vi "Set Convolution Kernel 32f.vi"(8 "Error In":errorcluster, 10 "Kernel In":sgl[][][](array[numeric]), 11 "Convolution Object":T1 {"Convolved Memory Object"."Dimension"."Width" min=1; "Convolved Memory Object"."Dimension"."Height" min=1; "Convolved Memory Object"."Dimension"."Depth" min=1; "Kernel Memory Object"."Dimension"."Width" min=1; "Kernel Memory Object"."Dimension"."Height" min=1; "Kernel Memory Object"."Dimension"."Depth" min=1}) -> (0 "Error Out":errorcluster, 3 "Convolution Object Out":T1 {"Convolved Memory Object"."Dimension"."Width" min=1; "Convolved Memory Object"."Dimension"."Height" min=1; "Convolved Memory Object"."Dimension"."Depth" min=1; "Kernel Memory Object"."Dimension"."Width" min=1; "Kernel Memory Object"."Dimension"."Height" min=1; "Kernel Memory Object"."Dimension"."Depth" min=1})   [LabVIEW 2012, in "OpenCLV x64.lvlib"]
doc: "Creates and copies a convolution kernel from Labview to the device. The convolution kernel should have have {N - 2, N - 2, N - 2} dimensions than the target memory being convolved."
uses:
  OpenCLV x64.lvlib
  Controls/Convolution Object.ctl
  Controls/Device ID.ctl
  Controls/Program Handle.ctl
  Controls/Memory Object.ctl
  Controls/Memory ID.ctl
  User Controls/Array Dimensions.ctl
  Controls/Memory Type.ctl
  Allocate Memory/AllocateMemory_32f.vi
  Write Memory/WriteMemory_32f.vi
  Error Checking/Add Error Functional Global.vi
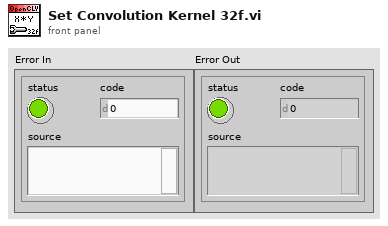
[diagram p1: front panel]
types:
  T1 = typedef "OpenCLV x64.lvlib/Convolution Object.ctl" = cluster{"Device In":T2, "Program Handle":T3, "Kernel Memory Object":T4, "Convolved Memory Object":T4}
  T2 = typedef "OpenCLV x64.lvlib/Device ID.ctl" = u64
  T3 = typedef "OpenCLV x64.lvlib/Program Handle.ctl" = u64
  T4 = typedef "OpenCLV x64.lvlib/Memory Object.ctl" = cluster{"Device ID":T2, "Memeroy ID":T5, "Dimension":T6, "Memory Type":T7}
  T5 = typedef "OpenCLV x64.lvlib/Memory ID.ctl" = u64
  T6 = typedef "Array Dimensions.ctl" = cluster{"Depth":u64, "Height":u64, "Width":u64}
  T7 = typedef "OpenCLV x64.lvlib/Memory Type.ctl" = enum16{"32f", "u8", "i8", "u16", "i16", "u32", "i32", "64f"}
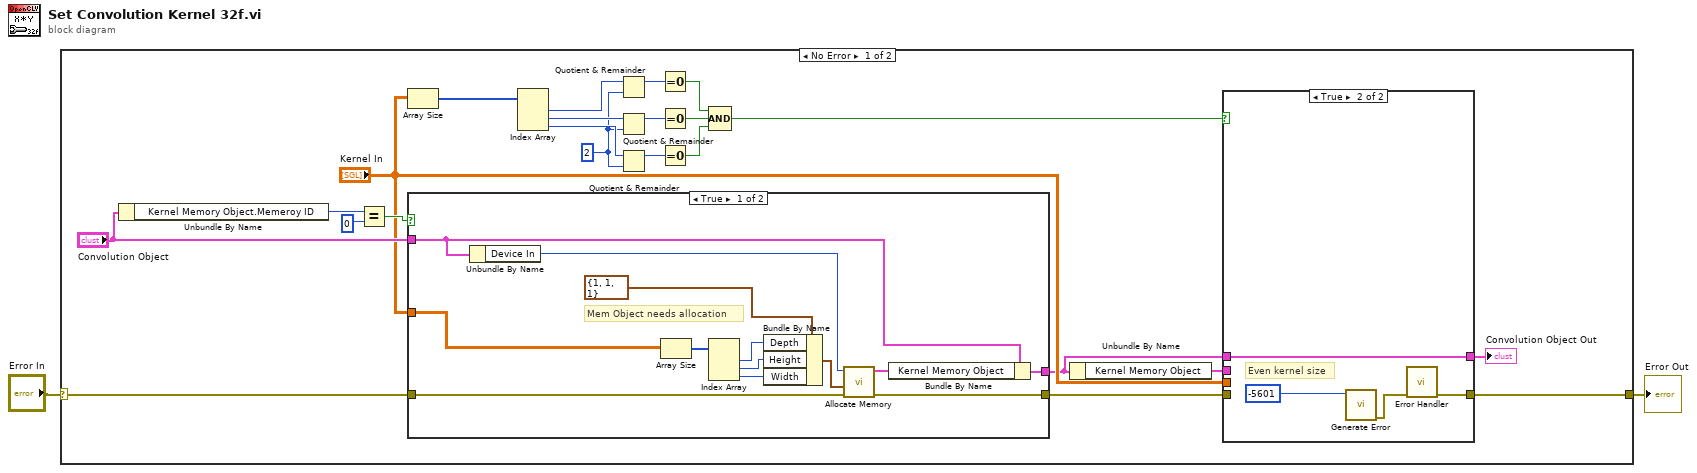
[diagram p0: block diagram]
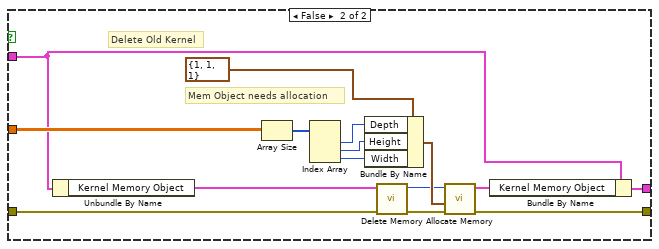
[diagram p2: hidden frame]
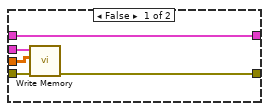
[diagram p3: hidden frame]
diagram:
  n1 = case shown="No Error" "Error In" {
    selector: "Error In" -> [w9 w63]
    tunnel: [w25 w63] -> w1
    frame No Error {
      w20 = 2 ("Argument Number")
      n2 = Unbundle By Name("Convolution Object") -> ("Kernel Memory Object.Memeroy ID"=w13:T5)
      n3 = Equal?(x=w13, y=T5 0) -> (x = y?=w11:bool)
      n4 = Array Size(array="Kernel In") -> (size(s)=w7:i32[])
      n5 = case shown="True" w11 {
        tunnel: "Convolution Object" -> [w28 w41]
        tunnel: w9 -> [w32 w44]
        tunnel: "Kernel In" -> [w31 w48]
        tunnel: [w29 w46] -> w8
        tunnel: [w26 w39] -> w4
        frame True {
          # "Mem Object needs allocation"
          n6 = Unbundle By Name(w28) -> ("Device In"=w38:T2)
          n7 = Array Size(array=w31) -> (size(s)=w30:i32[])
          n8 = Index Array(array=w30) -> (element #1=w33:i32, element #2=w34:i32, element #3=w35:i32)  [unwired: 3 in]
          n9 = Bundle By Name(cluster=T6 {"Depth"=1, "Height"=1, "Width"=1} ("Dimension"), "Depth"=w33, "Height"=w34, "Width"=w35) -> (w36:T6)
          n10 = call-poly "Allocate Memory.vi"("Error In"=w32, "Dimension"=w36, "Device In"=w38) -> ("Error Out"=w29:errorcluster, "Memory Object"=w27:T4)  [unwired: 6 in, 1 out]
          n11 = Bundle By Name(cluster=w28, "Kernel Memory Object"=w27) -> (w26:T1)
        }
        frame False {
          # "Delete Old Kernel"
          # "Mem Object needs allocation"
          n12 = Unbundle By Name(w41) -> ("Kernel Memory Object"=w42:T4)
          n13 = Array Size(array=w48) -> (size(s)=w47:i32[])
          n14 = Index Array(array=w47) -> (element #1=w49:i32, element #2=w50:i32, element #3=w51:i32)  [unwired: 3 in]
          n15 = Bundle By Name(cluster=T6 {"Depth"=1, "Height"=1, "Width"=1} ("Dimension"), "Depth"=w49, "Height"=w50, "Width"=w51) -> (w52:T6)
          n16 = call "Delete Memory.vi"("Error In"=w44, "Memory Object In"=w42) -> ("Error Out"=w43:errorcluster, "Device Out"=w45:T2)  [unwired: 8 in]
          n17 = call-poly "Allocate Memory.vi"("Error In"=w43, "Dimension"=w52, "Device In"=w45) -> ("Error Out"=w46:errorcluster, "Memory Object"=w40:T4)  [unwired: 6 in, 1 out]
          n18 = Bundle By Name(cluster=w41, "Kernel Memory Object"=w40) -> (w39:T1)
        }
      }
      n19 = Index Array(array=w7) -> (element #1=w14:i32, element #2=w22:i32, element #3=w21:i32)  [unwired: 3 in]
      n20 = Quotient & Remainder(x=w14, y=w20) -> (x-y*floor(x/y)=w24:i32)  [unwired: 1 out]
      n21 = Quotient & Remainder(x=w22, y=w20) -> (x-y*floor(x/y)=w23:i32)  [unwired: 1 out]
      n22 = Quotient & Remainder(x=w21, y=w20) -> (x-y*floor(x/y)=w19:i32)  [unwired: 1 out]
      n23 = Equal To 0?(x=w24) -> (x = 0?=w18:bool)
      n24 = Equal To 0?(x=w23) -> (x = 0?=w17:bool)
      n25 = Equal To 0?(x=w19) -> (x = 0?=w16:bool)
      n26 = Compound Arithmetic op=AND(w18, w17, w16) -> (w15:bool)
      n27 = Unbundle By Name(w4) -> ("Kernel Memory Object"=w5:T4)
      n28 = case shown="True" w15 {
        tunnel: w8 -> [w57 _]
        tunnel: w5 -> [w58 _]
        tunnel: [w56 w59] -> w25
        tunnel: "Kernel In" -> [w55 _]
        tunnel: w4 -> [w54 w61]
        tunnel: [w54 w61] -> w3
        frame False {
          n29 = call-poly "Write Memory.vi"("Error In"=w57, "Data In"=w55, "Memory Object In"=w58) -> ("Error Out"=w56:errorcluster)  [unwired: 6 in, 2 out]
        }
        frame True {
          # "Even kernel size"
          n30 = call "Generate Error.vi"("Error"=-5601) -> ("error out"=w60:errorcluster)  [unwired: 10 in]
          n31 = call-poly "Error Handler.vi"("Error In"=w60) -> ("Error Out"=w59:errorcluster)  [unwired: 10 in]
        }
      }
      "Convolution Object Out" <- w3
    }
    frame Error {
    }
  }
  "Error Out" <- w1
